vi "AudioTest, Audio Test Util, Parse Returned Data File.vi"(8 "error in (no error)":errorcluster, 11 "File Path":path) -> (1 "Desc":string, 2 "Numeric":i32, 3 "Result":T1)   [LabVIEW 2018]
uses:
  Functional Test/TypeDefs/FunctTest.Result State.ctl
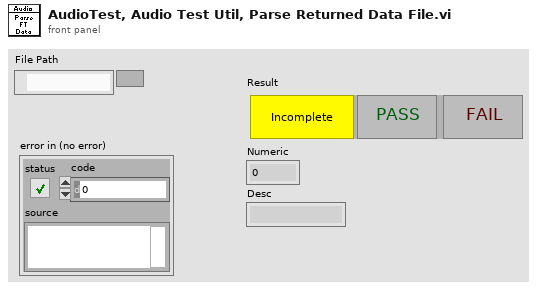
[diagram p1: front panel]
types:
  T1 = typedef "FunctTest.Result State.ctl" = enum32{"NoTest", "PASS", "FAIL"}
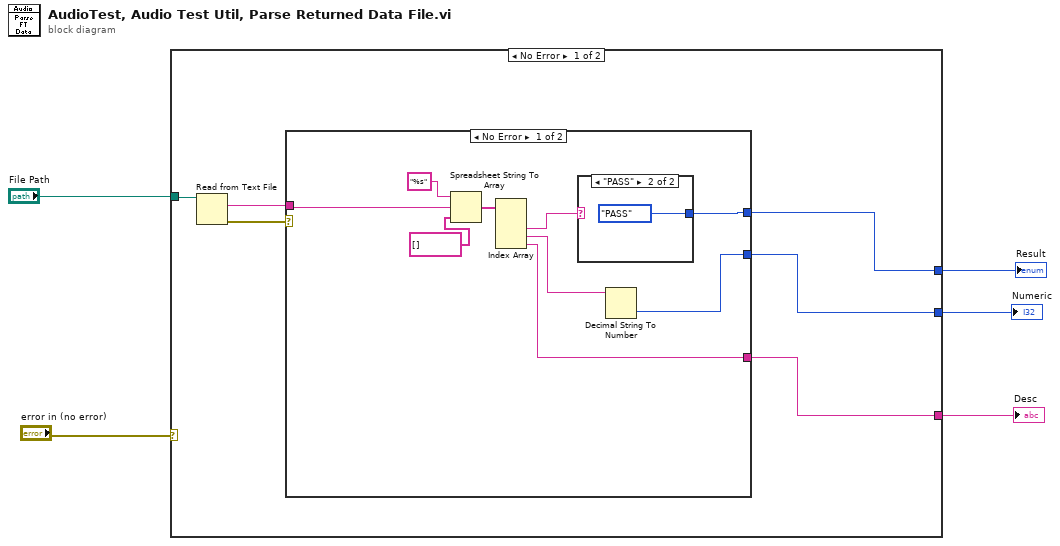
[diagram p0: block diagram]
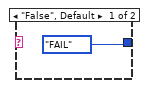
[diagram p2: hidden frame]
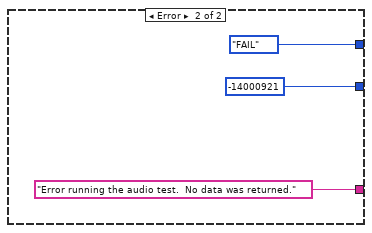
[diagram p3: hidden frame]
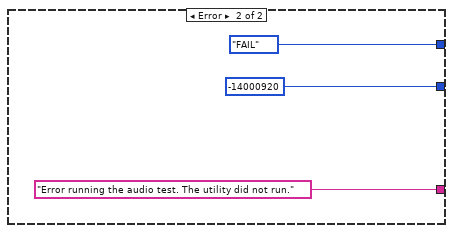
[diagram p4: hidden frame]
diagram:
  n1 = case shown="No Error" "error in (no error)" {
    tunnel: "File Path" -> [w11 _]
    tunnel: [w7 FunctTest.Result_State."FAIL" ("Result")] -> w4
    tunnel: [w8 -14000920] -> w3
    tunnel: [w6 "Error running the audio test. The utility did not run."] -> w2
    frame No Error {
      n2 = Read from Text File(file (use dialog)=w11) -> (text=w9:string, error out=w10:errorcluster)  [unwired: 3 in, 2 out]
      n3 = case shown="No Error" w10 {
        tunnel: w9 -> [w20 _]
        tunnel: [w13 -14000921] -> w8
        tunnel: [w15 FunctTest.Result_State."FAIL" ("Result")] -> w7
        tunnel: [w12 "Error running the audio test.  No data was returned."] -> w6
        frame No Error {
          n4 = Spreadsheet String To Array(format string="%s", spreadsheet string=w20, array type (2D Dbl)=string[] []) -> (array=w17:string[])  [unwired: 1 in]
          n5 = Index Array(array=w17) -> (element #2=w16:string, element #3=w14:string, element #4=w12:string)  [unwired: 4 in, 1 out]
          n6 = case shown="\"PASS\"" w16 {
            tunnel: [FunctTest.Result_State."FAIL" ("Result") FunctTest.Result_State."PASS" ("Result")] -> w15
            frame "False", Default {
            }
            frame "PASS" {
            }
          }
          n7 = Decimal String To Number(string=w14) -> (number=w13:i32)  [unwired: 2 in, 1 out]
        }
        frame Error {
        }
      }
    }
    frame Error {
    }
  }
  "Result" <- w4
  "Numeric" <- w3
  "Desc" <- w2
